vi "rt-test.vi"() -> ()   [LabVIEW 2020]
uses:
  Addon Engine/Types/FPGA Refnum.ctl
  <vilib>/Utility/error.llb/Error Cluster From Error Code.vi
  <vilib>/rvi/errors/niLvFpgaAdjustHostInterfaceError.vi
  <vilib>/xnet/xnet.llb/XNET Convert.vi
  <vilib>/xnet/xnet.llb/XNET Convert (Signal to Frame CAN).vi
  Addon Engine/SubVI/CAN Frames Write.vi
  Addon Engine/SubVI/CAN Frames Read.vi
  <vilib>/xnet/xnet.llb/XNET Convert (Frame CAN to Signal).vi
  <vilib>/FPGAPlugInAG/Dynamic/niLvFpga_Close_Dynamic.vi
  <vilib>/rvi/interface/nirviReadWriteControl/nirviReadWriteControl.xnode
  <vilib>/rvi/interface/nirviCloseFPGA/nirviCloseFPGA.xnode
  Addon Engine/985x Support Addon Engine.lvlib
  NiFpgaLv.dll
  <vilib>/rvi/interface/Simulation/niFpgaSimulationCallBeginRW.vi
panel:
  out "CAN1_Tx":u32[](array[numeric]) format="%.0x"
  out "CAN1_Rx":u32[](array[numeric]) format="%.0x"
  out "CAN0_Tx":u32[](array[numeric]) format="%.0x"
  out "CAN0_Rx":u32[](array[numeric]) format="%.0x"
  in  "CAN0":dbl[](array[numeric])=[1.0, 2.0] caption="signal data" format="%.2f"
  in  "Write":bool
  out "error out":errorcluster
  in  "stop":bool
  out "CAN1":dbl[](array[numeric]) caption="signal data" format="%.2f"
  in  "signal list":refnum<k21>[](array[refnum])=["CANEventSignal1\nNIXNET_example.CAN_Cluster", "CANCyclicSignal2\nnixnet_example.CAN_Cluster"]
  in  "Bitfile path":path=path "c:/ni-rt/VeriStand/Custom Devices/FPGA Addon/985xsupport_FPGATarget_fpga-main_5XgmTEdlmQU.lvbitx"
  in  "Device address":string="RIO0"
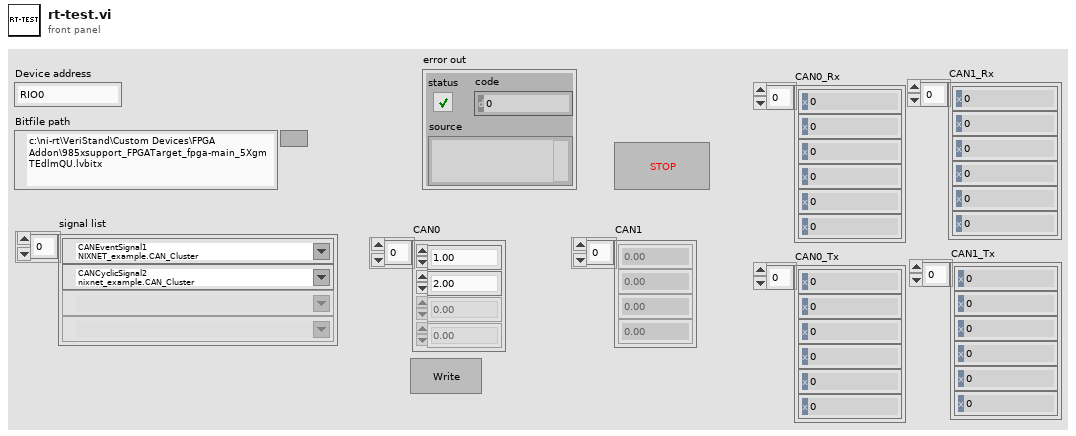
[diagram p1: front panel]
types:
  T1 = typedef "985x Support Addon Engine.lvlib/FPGA Refnum.ctl" = refnum<k20>
  T2 = typedef "985x Support Addon Engine.lvlib/Tx Event Session.ctl" = cluster{"FPGA Refnum":T1, "Channel Number":u32, "Conv Session":refnum<k21>}
  T3 = typedef "985x Support Addon Engine.lvlib/Rx Session.ctl" = cluster{"FPGA Refnum":T1, "Channel Number":u32, "Conv Session":refnum<k21>, "Signal ID":u32[], "Signals DVR":refnum<data-value>}
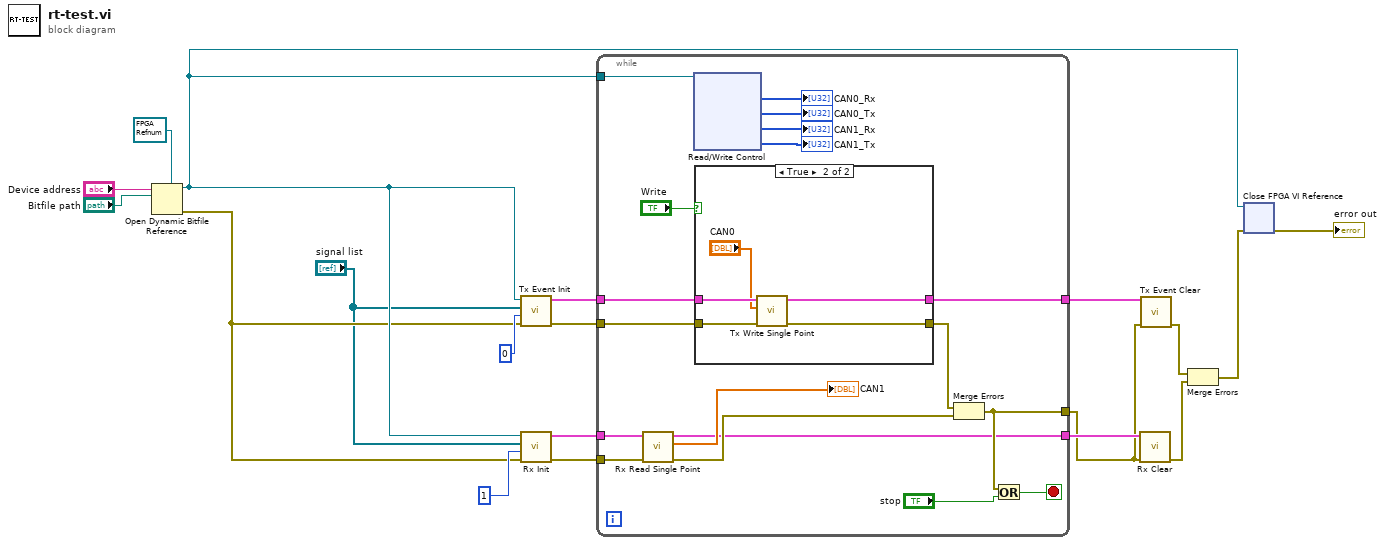
[diagram p0: block diagram]
diagram:
  n1 = Open Dynamic Bitfile Reference(0:"Device address", 1:"Bitfile path", 4:T1 refnum ("FPGA Refnum")) -> (5:w3:T1, 8:w2:errorcluster)  [unwired: 2 in]
  n2 = call "Tx Event Init.vi"("error in (no error)"=w2, "Channel Number"=u32 0, "signal list"="signal list", "FPGA Refnum"=w3) -> ("error out"=w12:errorcluster, "Tx Event"=w13:T2)  [unwired: 6 in]
  n3 = call "Rx Init.vi"("error in (no error)"=w2, "Channel Number"=u32 1, "signal list"="signal list", "FPGA Refnum"=w3) -> ("error out"=w18:errorcluster, "Rx Session"=w16:T3)  [unwired: 6 in]
  n4 = while {
    tunnel: [w35] -> w10
    tunnel: w18 -> [w34]
    tunnel: w16 -> [w30]
    tunnel: [w31] -> w17
    tunnel: w13 -> [w28]
    tunnel: w12 -> [w27]
    tunnel: [w26] -> w11
    tunnel: w3 -> [w24]
    stop <- w37 stop-if-true
    n5 = call "Rx Read Single Point.vi"("error in (no error)"=w34, "Rx Session In"=w30) -> ("error out"=w32:errorcluster, "Data"=→"CAN1":dbl[], "Rx Session Out"=w31:T3)  [unwired: 7 in]
    n6 = xnode "Read/Write Control"("FPGA VI Reference In"=w24) -> ("CAN0_Rx"=→"CAN0_Rx":u32[], "CAN0_Tx"=→"CAN0_Tx":u32[], "CAN1_Rx"=→"CAN1_Rx":u32[], "CAN1_Tx"=→"CAN1_Tx":u32[])  [unwired: 1 in, 2 out]
    n7 = case shown="True" "Write" {
      tunnel: w28 -> [w39 w44]
      tunnel: w27 -> [w38 w42]
      tunnel: [w39 w41] -> w26
      tunnel: [w38 w40] -> w25
      frame False {
      }
      frame True {
        n8 = call "Tx Write Single Point.vi"("error in (no error)"=w42, "Outgoing data"="CAN0", "Tx Event In"=w44) -> ("error out"=w40:errorcluster, "Tx Event Out"=w41:T2)  [unwired: 7 in]
      }
    }
    n9 = Merge Errors(w25, w32) -> (w35:errorcluster)
    n10 = Or(x=w35, y="stop") -> (x .or. y?=w37:bool)
  }
  n11 = call "Rx Clear.vi"("error in (no error)"=w10, "Rx Session In"=w17) -> ("error out"=w8:errorcluster)  [unwired: 9 in]
  n12 = call "Tx Event Clear.vi"("error in (no error)"=w10, "Tx Event"=w11) -> ("error out"=w9:errorcluster)  [unwired: 9 in]
  n13 = Merge Errors(w9, w8) -> (w7:errorcluster)
  n14 = xnode "Close FPGA VI Reference"("FPGA VI Reference In"=w3, "error in"=w7) -> ("error out"=→"error out":errorcluster)
